vi "Active Actor Monitor.vi"(7 "Write? (f)":bool, 10 "Monitor Type in":refnum<class "Actor Monitor.lvclass">) -> (2 "Monitor Type out":refnum<class "Actor Monitor.lvclass">)   [LabVIEW 2023, in "Monitored Actor.lvlib"]
doc: "Functional global that stores the type of actor monitor to use\n\nCopyright: MGI 2016\nAuthor: Derek Trepanier"
uses:
  Library/Monitored Actor.lvlib
  Actor Monitor/Actor Monitor/Actor Monitor.lvclass
  Classic Monitor/Monitor/Monitor Actor/Classic Monitor.lvclass
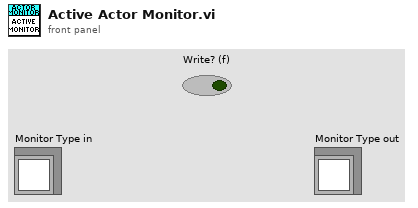
[diagram p1: front panel]
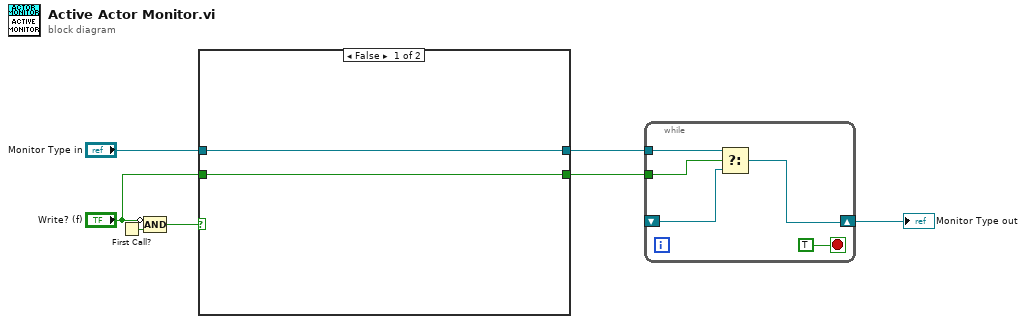
[diagram p0: block diagram]
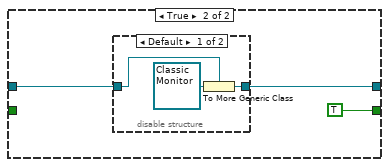
[diagram p2: hidden frame]
diagram:
  n1 = First Call?() -> (First Call?: T/F=w6:bool)
  n2 = Compound Arithmetic op=AND(invert "Write? (f)", w6) -> (w5:bool)
  n3 = case shown="False" w5 {
    tunnel: [w9 w11] -> w4
    tunnel: "Monitor Type in" -> [w9 w12]
    tunnel: [w8 TRUE] -> w2
    tunnel: "Write? (f)" -> [w8 _]
    frame False {
    }
    frame True {
      n4 = disable-structure shown="Default" {
        disable-tunnel: [w14 w16] -> w11
        disable-tunnel: w12 -> [w13 w16]
        frame condition #0 (active) {
          n5 = To More Generic Class(target class=w13, reference=refnum<class "Classic Monitor.lvclass"> refnum ("Classic Monitor.lvlib:Monitor.lvclass")) -> (generic class reference=w14:refnum<class "Actor Monitor.lvclass">)
        }
        frame condition #1 {
        }
      }
    }
  }
  n6 = while {
    tunnel: w4 -> [w20]
    tunnel: w2 -> [w19]
    shift-right: [w18] -> w7
    shift-left: _ -> [w17]
    stop <- TRUE stop-if-true
    n7 = Select(t=w20, s=w19, f=w17) -> (s? t:f=w18:refnum<class "Actor Monitor.lvclass">)
  }
  "Monitor Type out" <- w7
